vi "FitCoefficientsCalculationDynamicRange.vi"(10 "ArraySize":i32, 11 "FPGA VI Reference In":T3) -> (3 "FPGA VI Reference Out":T3)   [LabVIEW 2016]
uses:
  controls/FPGAVIreferenceTypeDef.ctl
  <vilib>/rvi/errors/niLvFpgaAdjustHostInterfaceError.vi
  <vilib>/Utility/error.llb/Error Cluster From Error Code.vi
  <vilib>/rvi/interface/nirviReadWriteControl/nirviReadWriteControl.xnode
  FPGA Bitfiles/qnmController797_usbRIO_controllerFPGAmu.lvbitx
  NiFpgaLv.dll
panel:
  out "Weights":T1(array[cluster])
  out "Coefficients":T2(array[cluster])
  in  "fitCoeffMin":i32=1
  in  "fitCoeffMax":i32=16
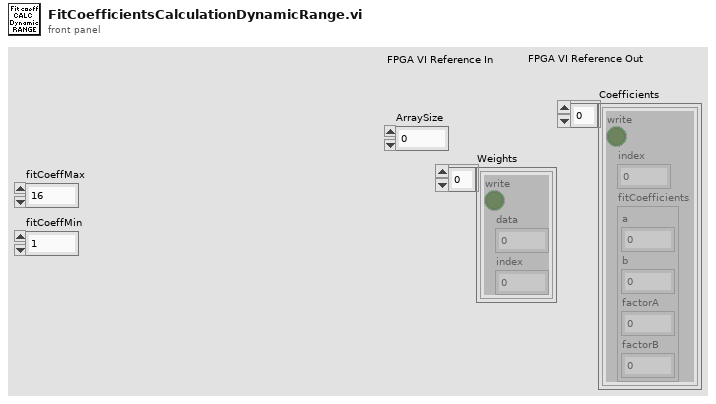
[diagram p1: front panel]
types:
  T1 = cluster{"write":bool, "data":fxp<+,20,0>, "index":u16}[]
  T2 = cluster{"write":bool, "index":u16, "fitCoefficients":cluster{"a":fxp<+/-,21,7>, "b":fxp<+/-,21,7>, "factorA":i8, "factorB":i8}}[]
  T3 = typedef "FPGAVIreferenceTypeDef.ctl" = refnum<k20>
  T4 = cluster{"write":bool, "index":u16, "fitCoefficients":cluster{"a":fxp<+/-,21,7>, "b":fxp<+/-,21,7>, "factorA":i8, "factorB":i8}}
  T5 = cluster{"write":bool, "data":fxp<+,20,0>, "index":u16}
  T6 = cluster{"a":fxp<+/-,21,7>, "b":fxp<+/-,21,7>, "factorA":i8, "factorB":i8}
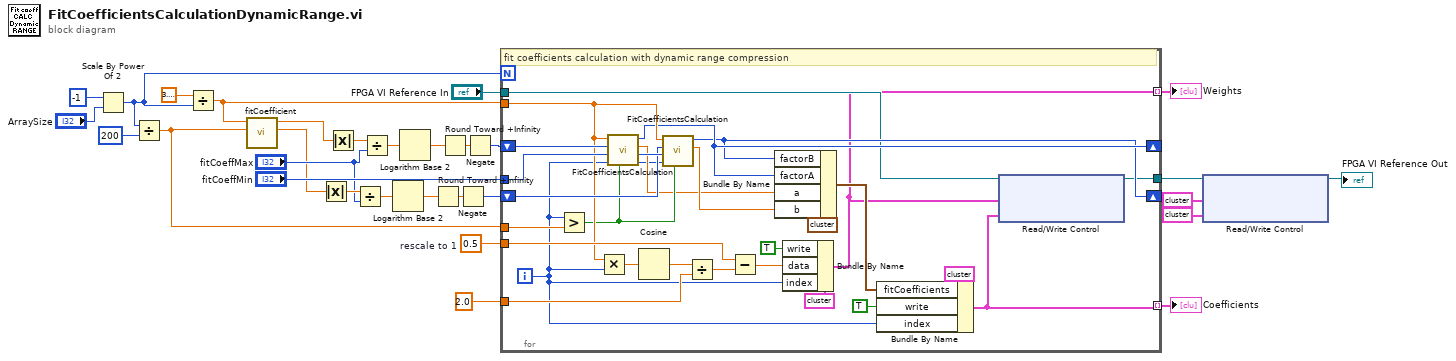
[diagram p0: block diagram]
diagram:
  w15 = 0.5  # rescale to 1
  n1 = Scale By Power Of 2(n=i16 -1, x="ArraySize") -> (x*2^n=w20:i32)
  n2 = Divide(x=w20, y=200) -> (x/y=w18:dbl)
  n3 = Divide(x=3.141592653589793, y=w20) -> (x/y=w29:dbl)
  n4 = call "fitCoefficient.vi"("n"=w18, "a"=w29) -> ("d"=w8:dbl, "c"=w28:dbl)  [unwired: 8 in]
  n5 = Absolute Value(x=w8) -> (abs(x)=w13:dbl)
  n6 = Absolute Value(x=w28) -> (abs(x)=w23:dbl)
  n7 = Divide(x=w13, y="fitCoeffMax") -> (x/y=w10:dbl)
  n8 = Divide(x=w23, y="fitCoeffMax") -> (x/y=w27:dbl)
  n9 = Logarithm Base 2(1:w10) -> (0:w11:dbl)
  n10 = Logarithm Base 2(1:w27) -> (0:w26:dbl)
  n11 = Round Toward +Infinity(x=w11) -> (ceil(x): smallest int >= x=w12:dbl)
  n12 = Round Toward +Infinity(x=w26) -> (ceil(x): smallest int >= x=w25:dbl)
  n13 = Negate(x=w12) -> (-x=w7:i16)
  n14 = Negate(x=w25) -> (-x=w22:i16)
  n15 = for {
    N: w20 -> [_]
    tunnel: w29 -> [w48]
    shift-right: [w37] -> _
    shift-left: w22 -> [w57]
    tunnel: "fitCoeffMin" -> [w50]
    tunnel: w18 -> [w56]
    tunnel: [w34] -> w4
    tunnel: 2.0 ("y") -> [w52]
    tunnel: w15 -> [w51]
    tunnel: "FPGA VI Reference In" -> [w35]
    shift-right: [w36] -> _
    shift-left: w7 -> [w49]
    tunnel: [w32] -> w2 mode=indexing
    tunnel: [w31] -> w1 mode=indexing
    i -> [w38]
    # "fit coefficients calculation with dynamic range compression"
    n16 = Greater?(x=w38, y=w56) -> (0:w47:bool)
    n17 = Multiply(x=w48, y=w38) -> (x*y=w55:dbl)
    n18 = call "FitCoefficientsCalculation.vi"("Iteration > 1/200*arraySize"=w47, "Iteration"=w38, "fitCoeffMin"=w50, "Numeric 4"=w57, "Pi/ArraySize"=w48) -> ("fitCoefficients.a-b"=w39:dbl, "fitCoefficients.Factor"=w37:i16)  [unwired: 5 in]
    n19 = Cosine(x=w55) -> (cos(x)=w54:dbl)
    n20 = call "FitCoefficientsCalculation.vi"("Iteration > 1/200*arraySize"=w47, "Iteration"=w38, "fitCoeffMin"=w50, "Numeric 4"=w49, "Pi/ArraySize"=w48) -> ("fitCoefficients.a-b"=w40:dbl, "fitCoefficients.Factor"=w36:i16)  [unwired: 5 in]
    n21 = Divide(x=w54, y=w52) -> (x/y=w53:dbl)
    n22 = Subtract(x=w51, y=w53) -> (x-y=w44:dbl)
    n23 = Bundle By Name(cluster=T6 {"a"=0.0, "b"=0.0, "factorA"=0, "factorB"=0} ("fitCoefficients"), "factorB"=w36, "factorA"=w37, "a"=w39, "b"=w40) -> (w33:T6)
    n24 = Bundle By Name(cluster=T5 {"write"=FALSE, "data"=0.0, "index"=0} ("ort.fit.m.weights"), "write"=TRUE, "data"=w44, "index"=w38) -> (w31:T5)
    n25 = Bundle By Name(cluster=T4 {"write"=FALSE, "index"=0, "fitCoefficients"={"a"=0.0, "b"=0.0, "factorA"=0, "factorB"=0}} ("ort.fit.m.coefficients"), "fitCoefficients"=w33, "write"=TRUE, "index"=w38) -> (w32:T4)
    n26 = xnode "Read/Write Control"("FPGA VI Reference In"=w35, "ort.fit.m.weights"=w31, "ort.fit.m.coefficients"=w32) -> ("FPGA VI Reference Out"=w34:T3)  [unwired: 1 in, 1 out]
  }
  "Coefficients" <- w2
  "Weights" <- w1
  n27 = xnode "Read/Write Control"("FPGA VI Reference In"=w4, "ort.fit.m.weights"=T5 {"write"=FALSE, "data"=0.0, "index"=0} ("fitWeightsWrite"), "ort.fit.m.coefficients"=T4 {"write"=FALSE, "index"=4, "fitCoefficients"={"a"=0.0, "b"=0.0, "factorA"=0, "factorB"=0}} ("fitFactorWrite")) -> ("FPGA VI Reference Out"=→"FPGA VI Reference Out":T3)  [unwired: 1 in, 1 out]
